vi "WriteMapping.vi"(8 "error in (no error)":errorcluster, 9 "TestCaseMap":map{string, set{string}}(c390), 10 "RequirementMap":map{string, set{string}}(c390), 11 "Pips in":refnum<class "Pips.lvclass">) -> (0 "error out":errorcluster, 3 "Pips out":refnum<class "Pips.lvclass">)   [LabVIEW 2021, in "Bananas.lvlib" / "Pips.lvclass"]
uses:
  Pips.lvclass
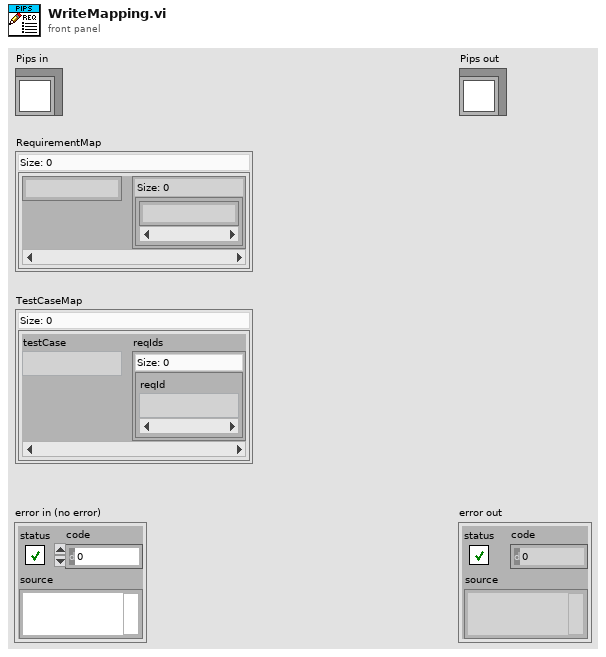
[diagram p1: front panel]
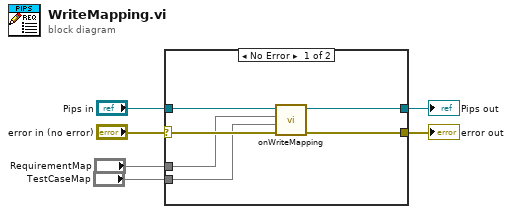
[diagram p0: block diagram]
diagram:
  n1 = case shown="No Error" "error in (no error)" {
    selector: "error in (no error)" -> [w11 w14]
    tunnel: [w8 w14] -> w5
    tunnel: [w9 w13] -> w3
    tunnel: "Pips in" -> [w12 w13]
    tunnel: "RequirementMap" -> [w10 _]
    tunnel: "TestCaseMap" -> [w7 _]
    frame No Error {
      n2 = call-dynamic "onWriteMapping.vi"("error in (no error)"=w11, "TestCaseMap"=w7, "RequirementMap"=w10, "Pips in"=w12) -> ("error out"=w8:errorcluster, "Pips out"=w9:refnum<class "Pips.lvclass">)  [unwired: 6 in]
    }
    frame Error {
    }
  }
  "error out" <- w5
  "Pips out" <- w3
